vi "Station_Meteo.vi"() -> ()   [LabVIEW 2018]
uses:
  <vilib>/Instr/_visa.llb/VISA Configure Serial Port (Instr).vi
panel:
  out "Temperature":string
  out "Humidity":string
  out "Pressure":string
  in  "Nom de ressource VISA":refnum<visa-resource-name>
  in  "stop":bool
  out "Chaîne":string
  # "1. Brancher la carte Arduino sur un port USB\n2. Choisir le port COM de la carte dans la liste déroulante \"Nom de ressource VISA\"\n3. Lancer le programme"
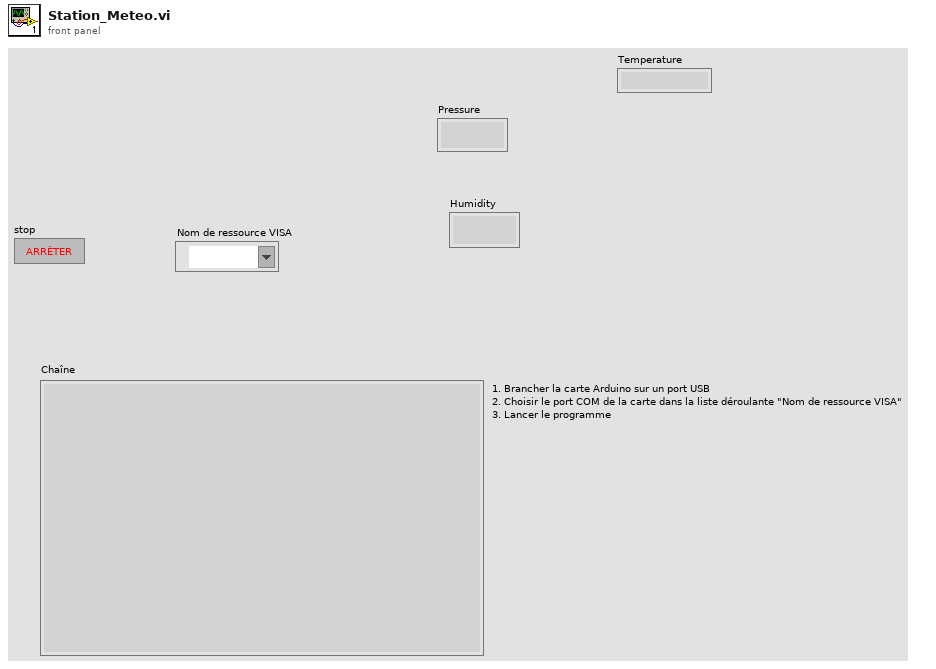
[diagram p1: front panel]
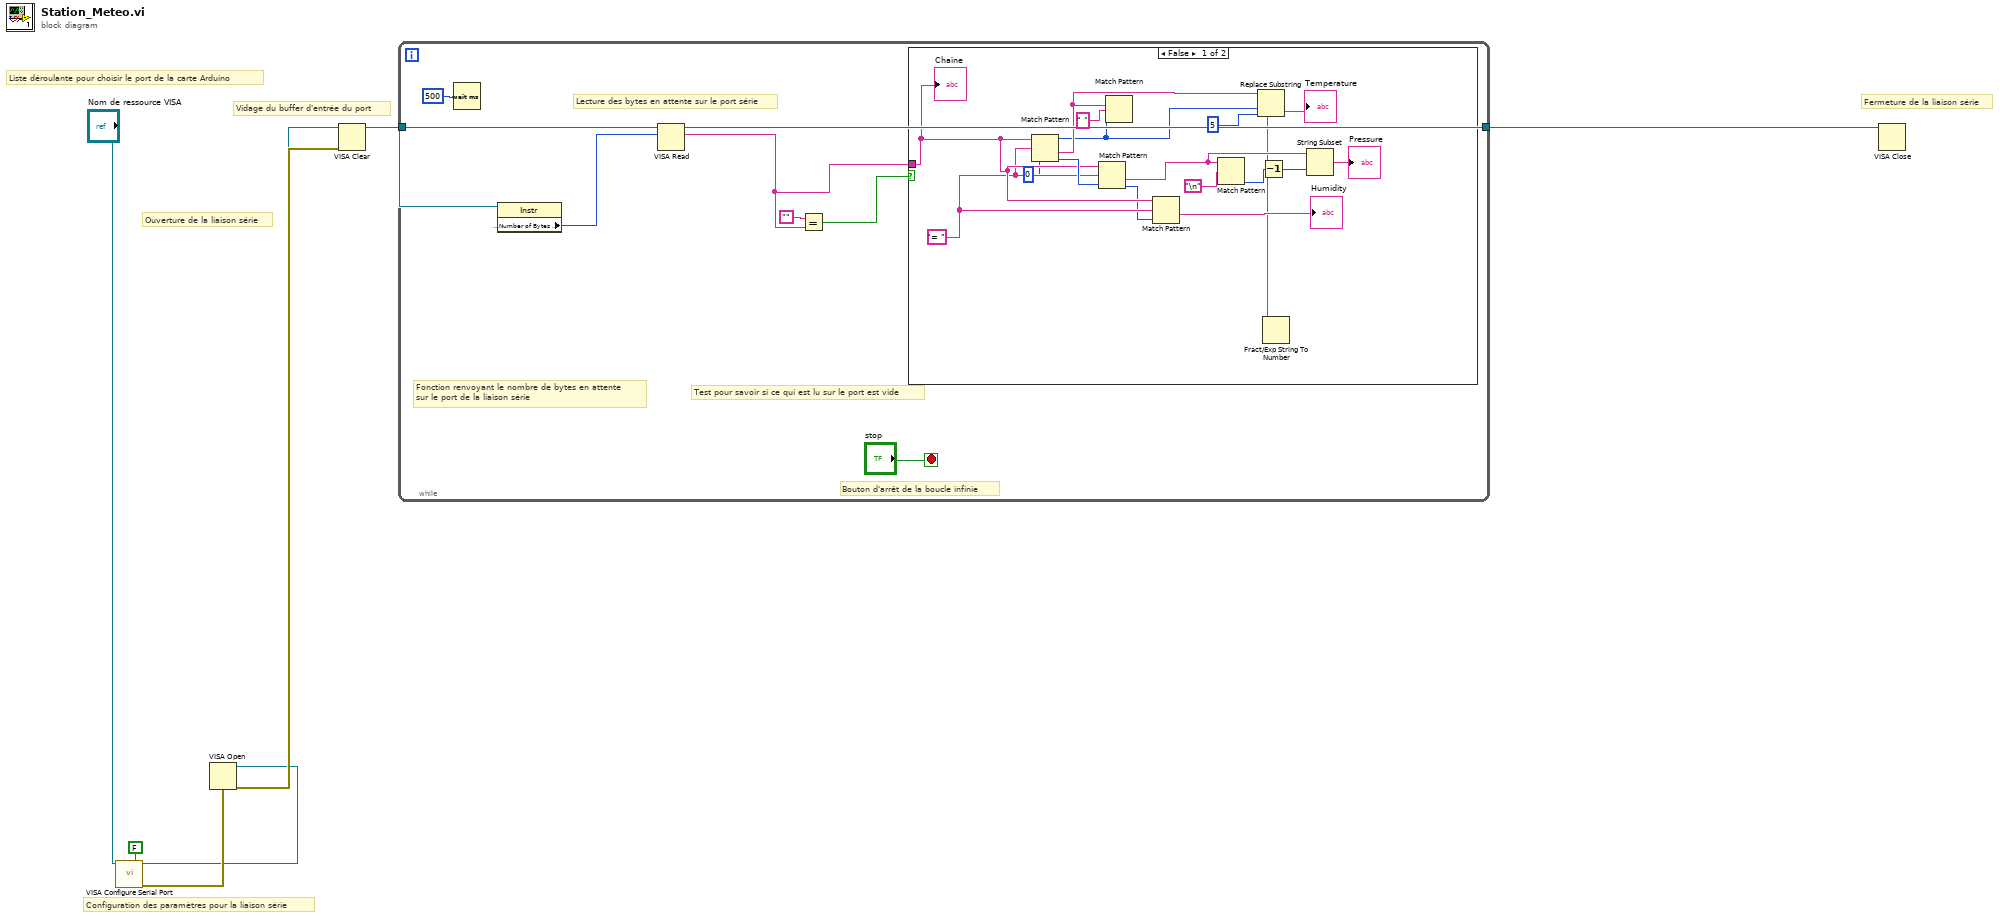
[diagram p0: block diagram]
diagram:
  # "Vidage du buffer d'entrée du port"
  # "Ouverture de la liaison série"
  # "Configuration des paramètres pour la liaison série"
  # "Liste déroulante pour choisir le port de la carte Arduino"
  # "Fermeture de la liaison série"
  n1 = call-poly "VISA Configure Serial Port"("VISA resource name"="Nom de ressource VISA", "Enable Termination\nChar (T)"=FALSE ("Enable Termination\nChar (T)")) -> ("VISA resource name out"=w4:refnum<visa-resource-name>, "error out"=w6:errorcluster)  [unwired: 12 in]
  n2 = VISA Open(error in (no error)=w6, VISA resource name=w4) -> (VISA resource name=w2:refnum<visa-resource-name>, error out=w7:errorcluster)  [unwired: 3 in]
  n3 = VISA Clear(VISA resource name=w2, error in (no error)=w7) -> (VISA resource name out=w3:refnum<visa-resource-name>)  [unwired: 1 out]
  n4 = while {
    tunnel: w3 -> [w15]
    tunnel: [w13] -> w8
    stop <- "stop" stop-if-true
    # "Lecture des bytes en attente sur le port série"
    # "Fonction renvoyant le nombre de bytes en attente\nsur le port de la liaison série"
    # "Test pour savoir si ce qui est lu sur le port est vide"
    # "Bouton d'arrêt de la boucle infinie"
    n5 = Wait (ms)(milliseconds to wait=u32 500 ("attente (ms)")) -> ()  [unwired: 1 out]
    n6 = property class="Instr"(reference=w15) -> ("Serial Settings:Number of Bytes at Serial Port"=w14:u32)  [unwired: 1 in, 2 out]
    n7 = VISA Read(VISA resource name=w15, byte count=w14) -> (VISA resource name out=w13:refnum<visa-resource-name>, read buffer=w9:string)  [unwired: 1 in, 2 out]
    n8 = Equal?(x="", y=w9) -> (x = y?=w10:bool)
    n9 = case shown="False" w10 {
      tunnel: w9 -> [w30 _]
      frame False {
        w19 = 0 ("offset (0)")
        w29 = "= " ("regular expression")
        n10 = Match Pattern(string=w30, regular expression=w29, offset (0)=w19) -> (after substring=w21:string, offset past match=w31:i32)  [unwired: 2 out]
        n11 = Match Pattern(string=w30, regular expression=w29, offset (0)=w31) -> (after substring=w25:string, offset past match=w26:i32)  [unwired: 2 out]
        n12 = Match Pattern(string=w21, regular expression=" ", offset (0)=w19) -> ()  [unwired: 4 out]
        n13 = Match Pattern(string=w30, regular expression=w29, offset (0)=w26) -> (after substring=→"Humidity":string)  [unwired: 3 out]
        n14 = Match Pattern(string=w25, regular expression="\n") -> (offset past match=w23:i32)  [unwired: 1 in, 3 out]
        n15 = Replace Substring(2:5 ("length (len. of substring)"), 3:w19, 5:w21) -> (0:w17:string)  [unwired: 1 in, 1 out]
        "Temperature" <- w17
        n16 = Decrement(x=w23) -> (x-1=w24:i32)
        n17 = Fract/Exp String To Number(string=w17) -> ()  [unwired: 3 in, 2 out]
        n18 = String Subset(string=w25, length (rest)=w24) -> (substring=→"Pressure":string)  [unwired: 1 in]
        "Chaîne" <- w30
      }
      frame True {
      }
    }
  }
  n19 = VISA Close(VISA resource name=w8) -> ()  [unwired: 1 in, 1 out]
